vi "data_analysis main.vi"() -> ()   [LabVIEW 2017]
uses:
  <vilib>/Analysis/baseanly.llb/Mean (DBL).vi
  <vilib>/Waveform/WDTFileIO.llb/Export Waveforms To Spreadsheet File (1D).vi
  <vilib>/Utility/file.llb/Read Delimited Spreadsheet (DBL).vi
  <vilib>/Analysis/NI_AALBase.lvlib
panel:
  out "size(Zmag)":i32
  out "size(Z)":i32
  in  "停止":bool
  out "Zmag trajectory":waveform(dbl) caption="元素"
  out "Ext.":dbl
  out "Z pos":waveform(dbl)[](graph)
  out "Zmag pos":waveform(dbl)(graph)
  out "data name":string
  out "cursor pos":dbl
  out "cursor length":dbl
  out "zmag cursor pos":dbl
  out "zmag cursor length":dbl
  out "current bead":string
  in  "graphs":enum32{"raw data", "force calculation"}(tab)
  in  "next":bool
  out "XY图":cluster{dbl[], dbl[]}(graph)
  in  "ref NO.":i32 min=0
  in  "remove drift":bool
  in  "sample rate":dbl=200.0
  in  "zero point offset":bool
  out "x_0":dbl caption="X0" format="%0.2f"
  out "y_0":dbl caption="Y0" format="%0.2f"
  out "z_0":dbl caption="Z0" format="%0.2f"
  in  "file save path":path
  in  "数据另存为":bool
  in  "data type":enum16{"tdms", "gr", "excel"}(ring)
  out "保存完成？":bool
  in  "file path":path
  in  "load data":bool
  in  "data info":i32(listbox)
  in  "bead NO.":i32 min=0
  in  "trajectory":i32 min=0
  out "Z mag":dbl
  in  "zmag or force":enum32{"zmag", "force"}(radio)
  in  "load txt":bool
  out "data num":i32
  in  "Last":bool
  out "size(align)":i32
  in  "left rank":i32=10
  in  "right rank":i32=8
  in  "doubleFace?":bool
  in  "B":dbl=-1.436
  in  "A":dbl=142.6
  in  "cali source":enum32{"X", "Y"}(radio)
  out "Power spectrum (um^2/Hz)":cluster{dbl[], "Spectrum out":dbl[]}[](graph)
  in  "Z_shift":dbl
  out "Force graph":cluster{dbl[], dbl[]}(graph)
  in  "accept":bool
  in  "force estimate":bool
  in  "Fit settings":T1={"#PSD Averages"=40, "Correct camera acquisition artifacts"=TRUE, "Autorange"=TRUE, "fstart (Hz)"=0.0, "Pendulum geometry"=FALSE, "Fit model"=FALSE} {"#PSD Averages" min=1}
  in  "fsampling (Hz)":dbl=2800.0
  in  "DNA length (um)":dbl=0.658
  out "Fit Results":T2
  out "fit data":dbl[][](array[numeric])
  # "load force-zmag"
  # "F="
  # "exp(                *Zmag)"
  # "*"
  # "exp(                *Zmag)"
  # "+"
  # "*"
  # "Fit parameters"
  # "Calculated quantities"
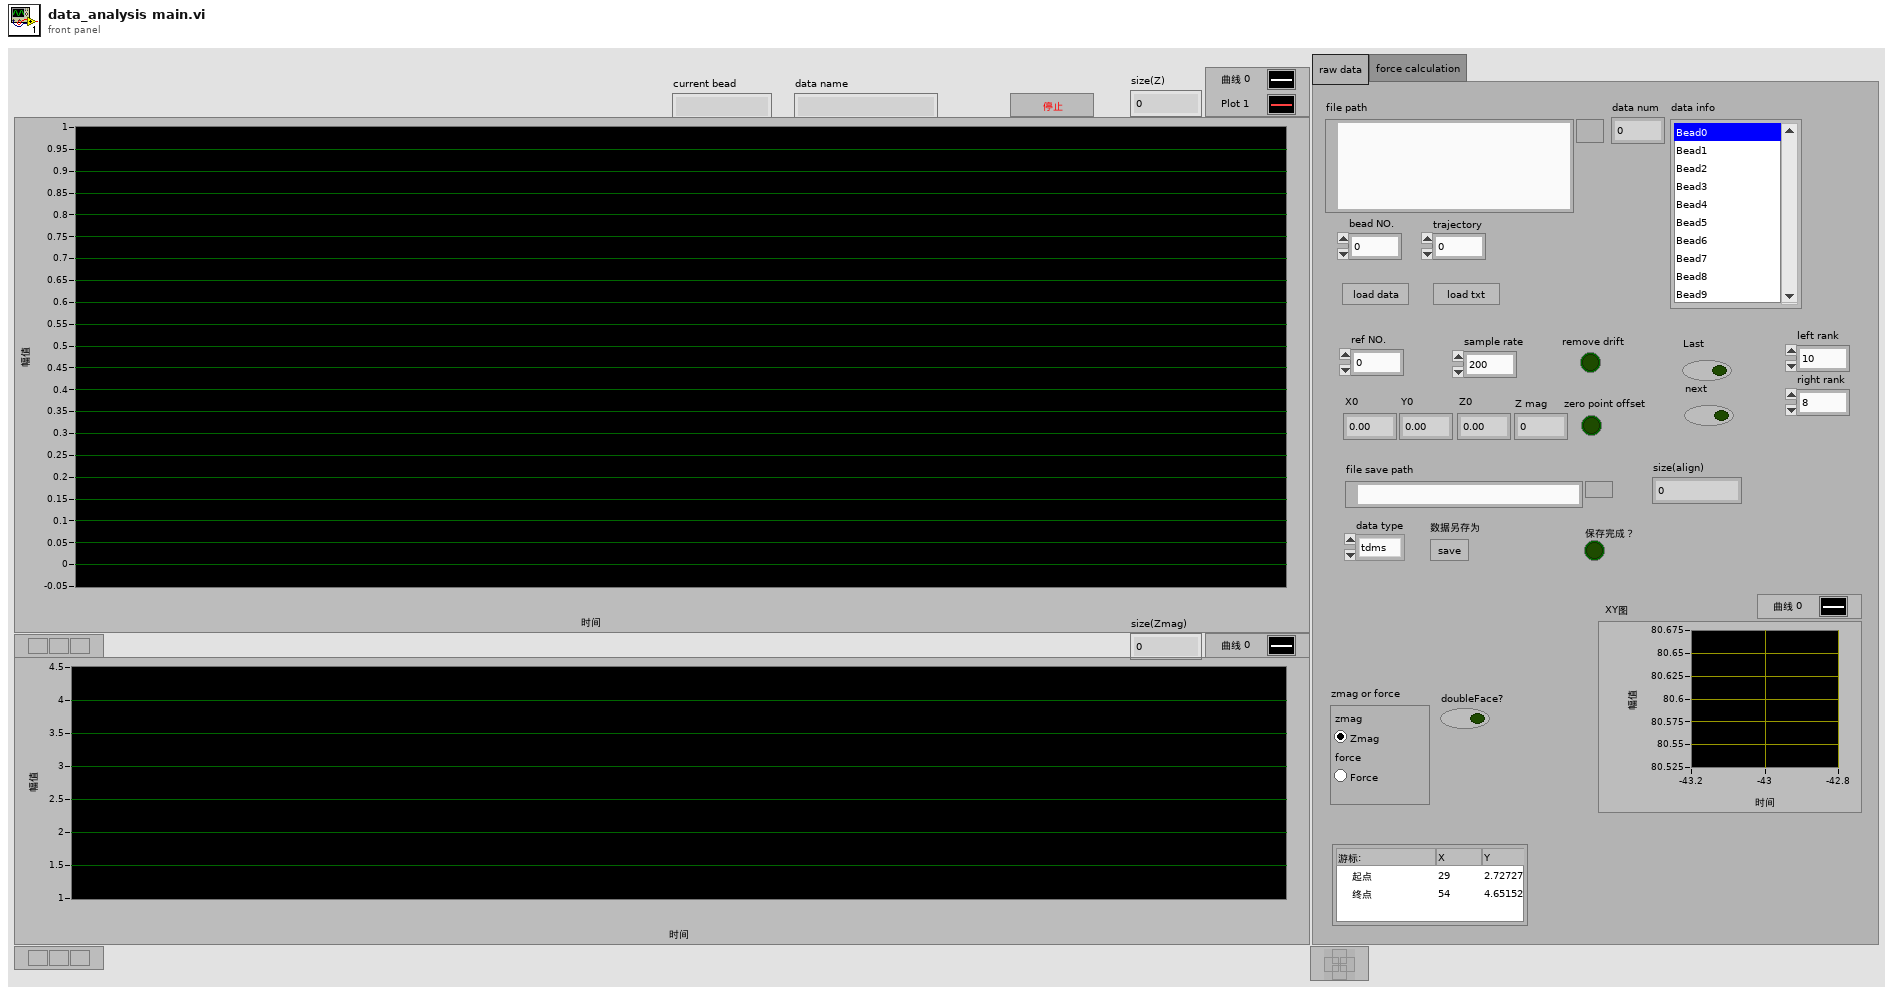
[diagram p1: front panel]
types:
  T1 = cluster{"#PSD Averages":u8, "Correct camera acquisition artifacts":bool, "Autorange":bool, "fstart (Hz)":dbl, "Pendulum geometry":bool, "Fit model":bool}
  T2 = cluster{"fcut (Hz)":dbl, "x2 (µm^2)":dbl, "Force (pN)":dbl, "Radius (µm)":dbl, "Apparent hydrodyn. radius (µm)":dbl, "fcut Error (Hz)":dbl, "x2 Error (µm^2)":dbl, "Force Error (pN)":dbl, "Radius Error (µm)":dbl, "Residue (unbiased)":dbl, "In range?":bool}
  T3 = enum16{"open", "open or create", "create or replace", "create", "open (read-only)"}
  T4 = enum16{"big-endian, network order", "native, host order", "little-endian"}
  T5 = enum16{"open", "replace", "create", "open or create", "replace or create", "replace or create with confirmation"}
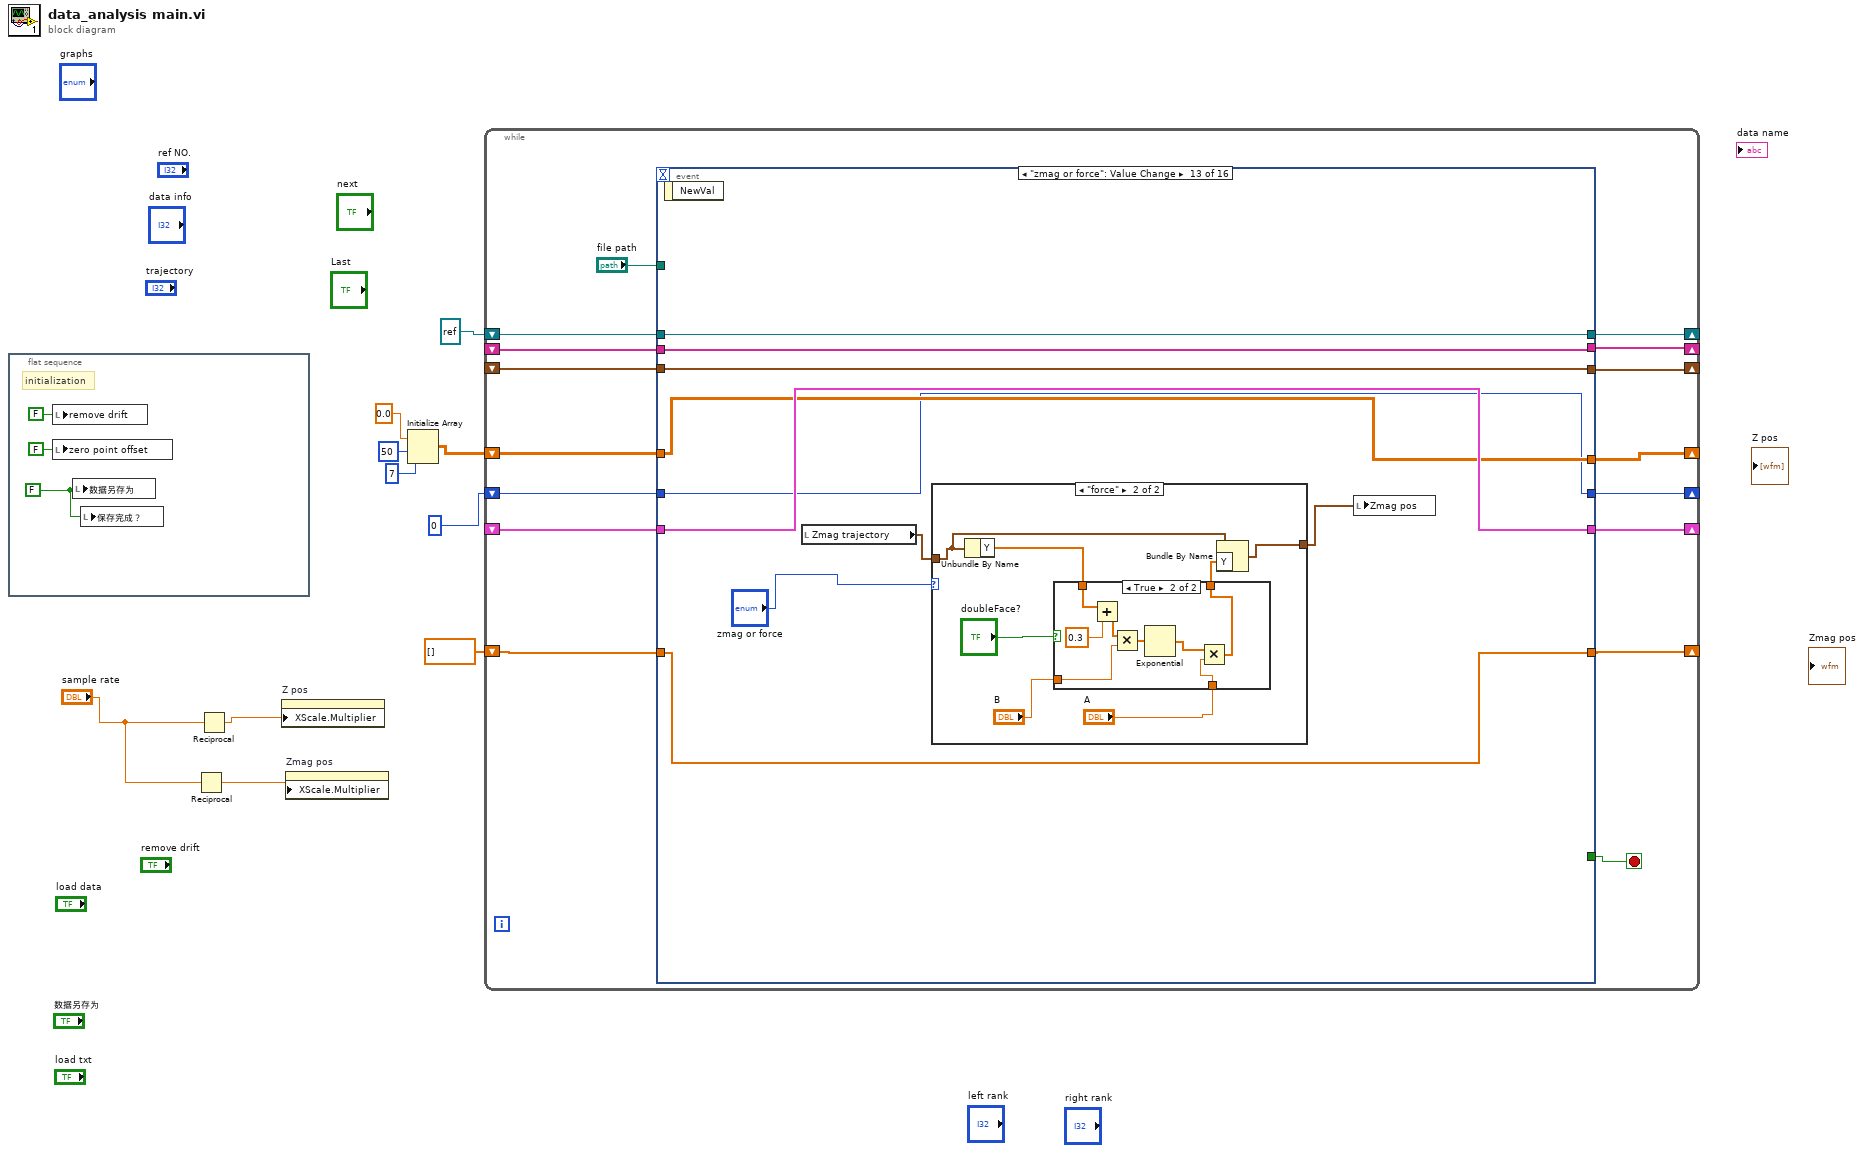
[diagram p0: block diagram]
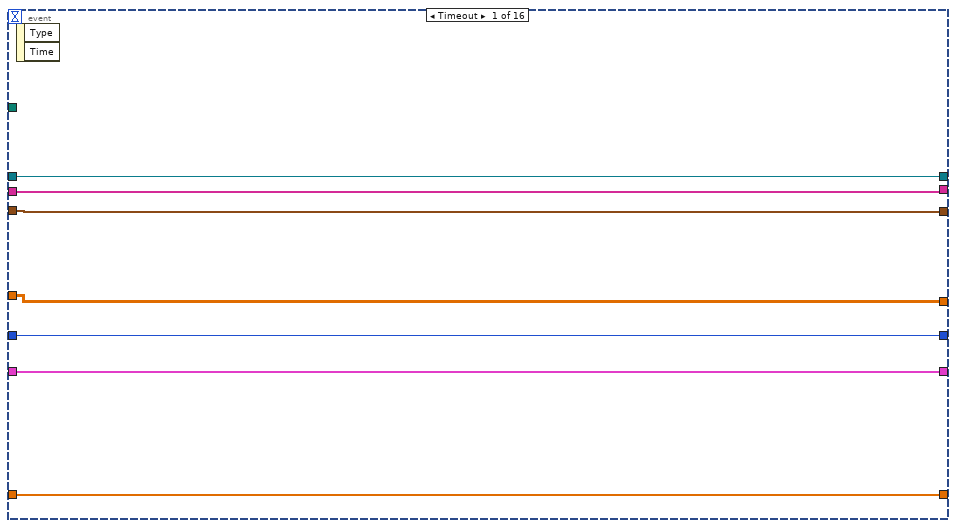
[diagram p2: hidden frame]
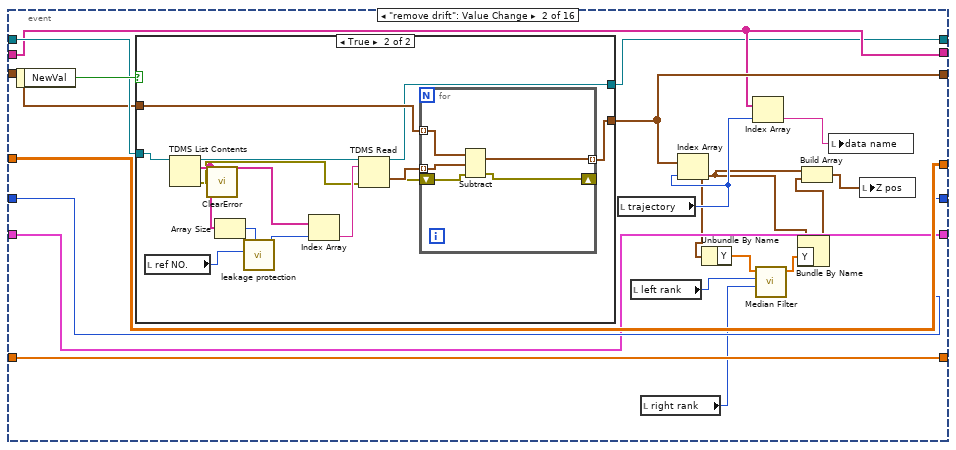
[diagram p3: hidden frame]
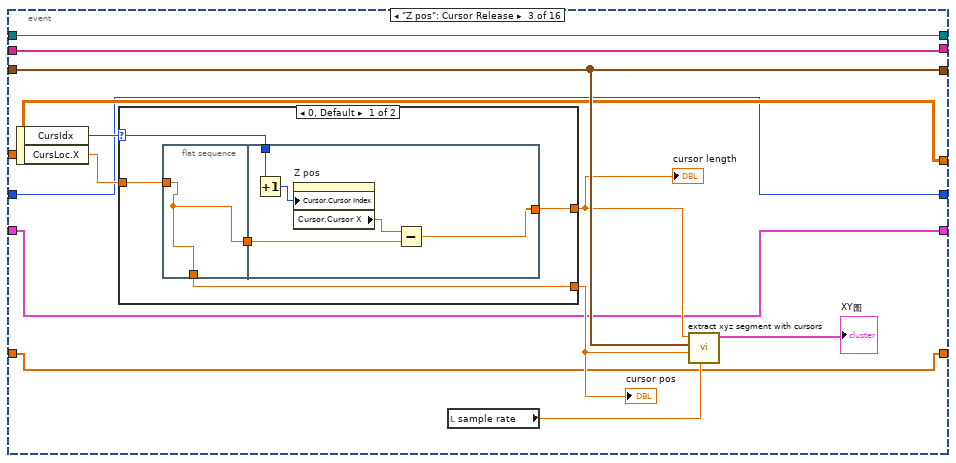
[diagram p5: hidden frame]
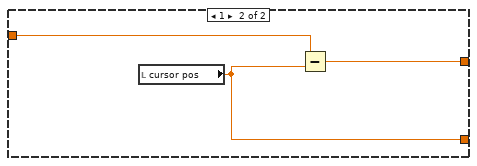
[diagram p6: hidden frame]
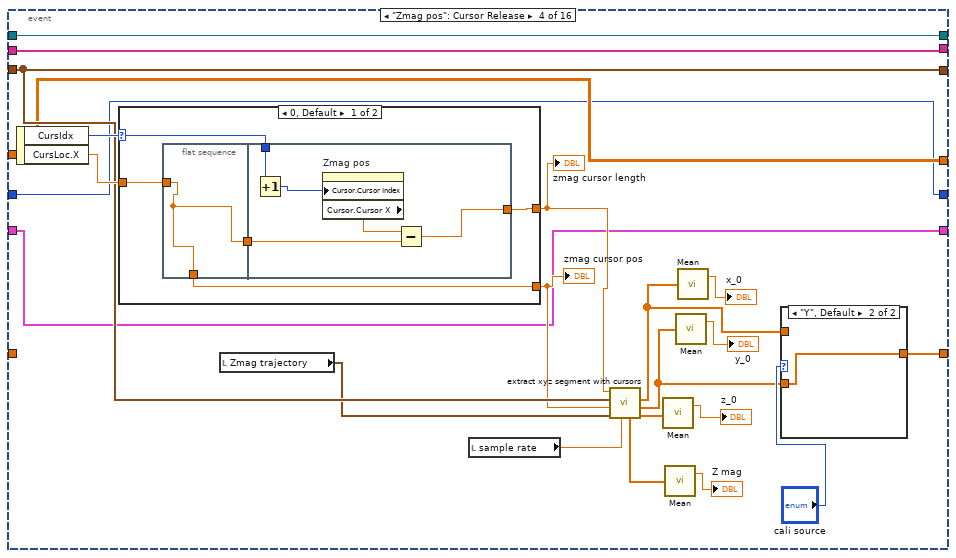
[diagram p7: hidden frame]
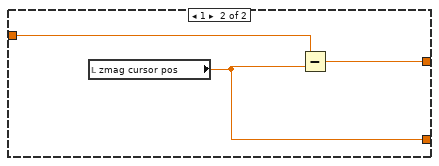
[diagram p9: hidden frame]
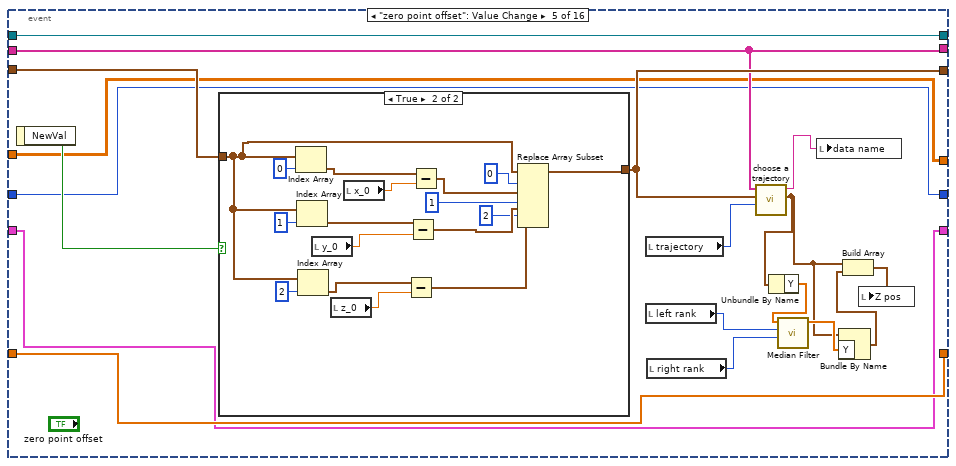
[diagram p10: hidden frame]
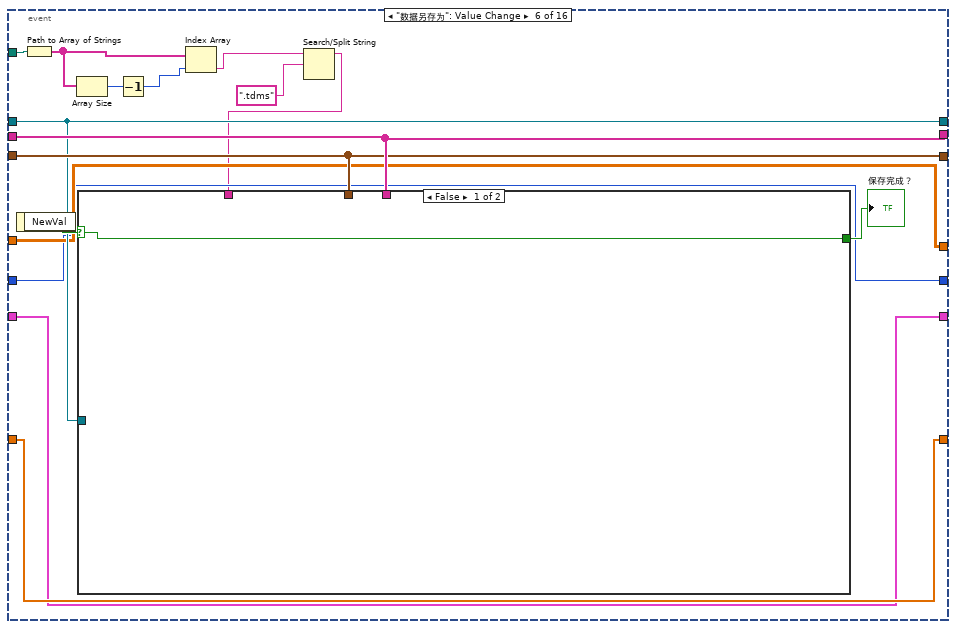
[diagram p12: hidden frame]
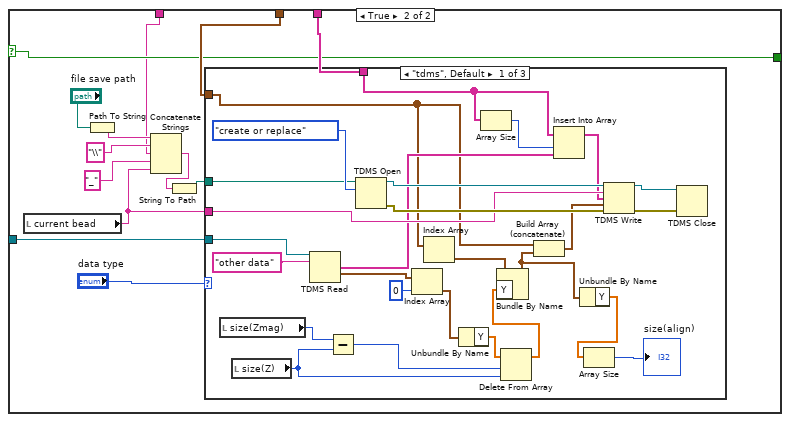
[diagram p13: hidden frame]
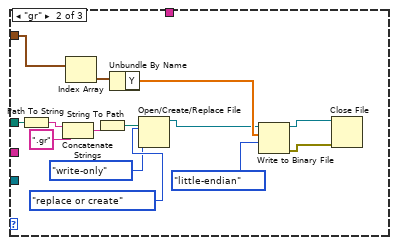
[diagram p14: hidden frame]
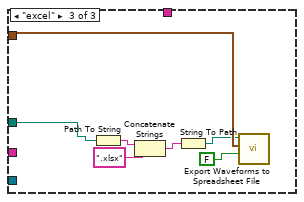
[diagram p15: hidden frame]
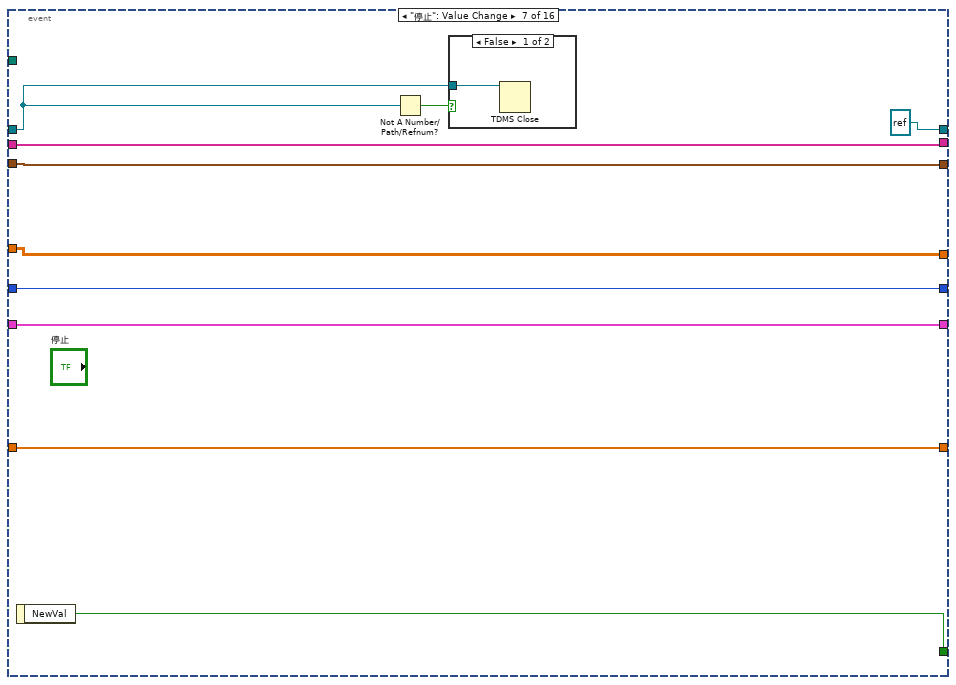
[diagram p16: hidden frame]
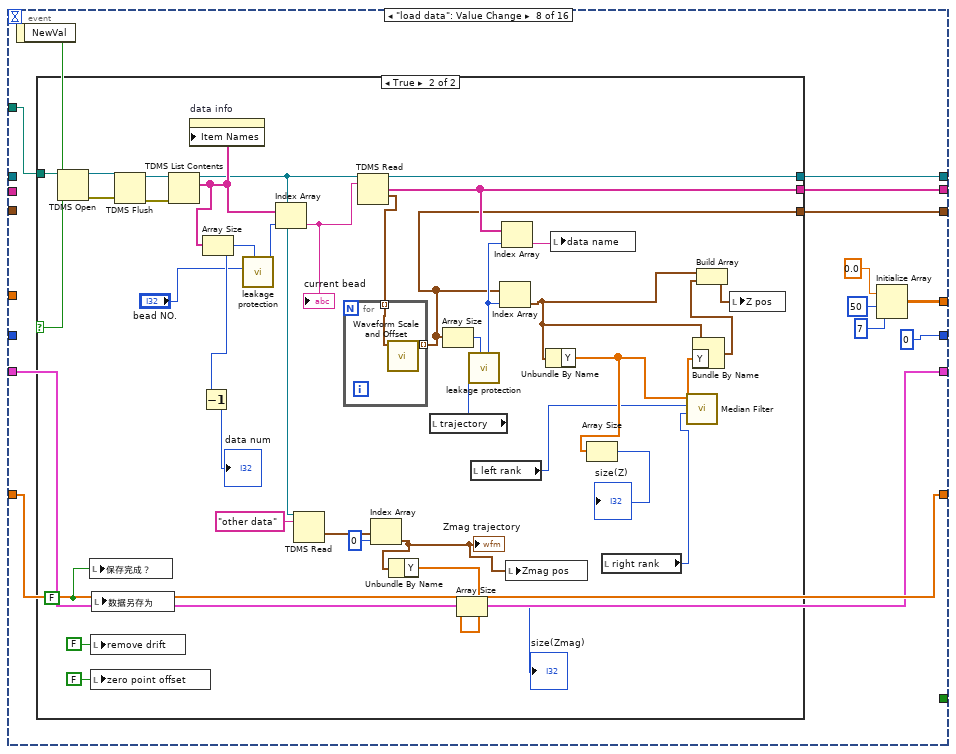
[diagram p18: hidden frame]
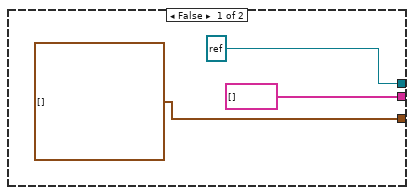
[diagram p19: hidden frame]
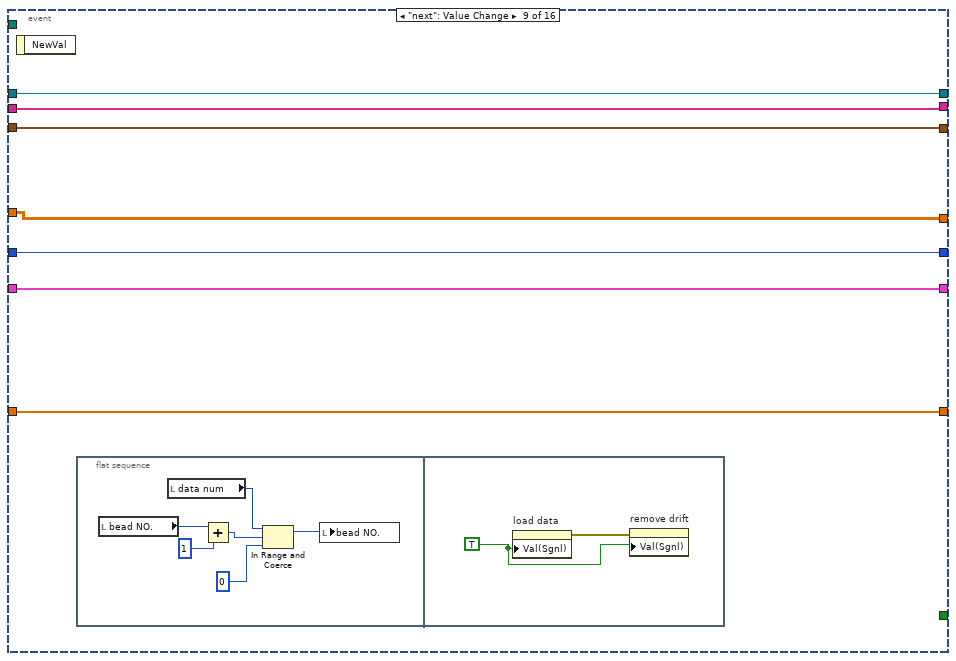
[diagram p20: hidden frame]
diagram:
  n1 = flat-sequence {
    frame #0 {
      w11 = FALSE ("数据另存为")
      # "initialization"
      n2 = local write "remove drift"(FALSE ("remove drift")) -> ()
      n3 = local write "zero point offset"(FALSE ("zero point offset")) -> ()
      n4 = local write "数据另存为"(w11) -> ()
      n5 = local write "保存完成？"(w11) -> ()
    }
  }
  n6 = Reciprocal(x="sample rate") -> (1/x=w1:dbl)
  n7 = Reciprocal(x="sample rate") -> (1/x=w3:dbl)
  n8 = property on="Z pos" class="WFGraph (strict)"("XScale.Multiplier"=w3) -> ()  [unwired: 2 in, 2 out]
  n9 = property on="Zmag pos" class="WFGraph (strict)"("XScale.Multiplier"=w1) -> ()  [unwired: 2 in, 2 out]
  n10 = Initialize Array(0.0 ("元素"), 50 ("维数大小"), 7 ("维数大小")) -> (w7:dbl[][])
  n11 = while {
    shift-right: [w27] -> _
    shift-left: refnum<k34> refnum ("tdms file out") -> [w22]
    shift-right: [w26] -> _
    shift-left: _ -> [w24]
    shift-right: [w25] -> _
    shift-left: _ -> [w23]
    shift-right: [w21] -> _
    shift-left: dbl[] [] ("Y") -> [w20]
    shift-right: [w19] -> _
    shift-left: _ -> [w18]
    shift-right: [w15] -> _
    shift-left: w7 -> [w17]
    shift-right: [w14] -> _
    shift-left: 0 -> [w16]
    stop <- w29 stop-if-true
    n12 = event "事件结构" shown="[12] \"zmag or force\": Value Change" {
      selector: _ -> [_ _ _ _ _ _ _ _ _ _ _ _ _ _ _ _]
      dyn-events: _ -> [_ _ _ _ _ _ _ _ _ _ _ _ _ _ _ _]
      timeout: _ -> [_ _ _ _ _ _ _ _ _ _ _ _ _ _ _ _]
      tunnel: [_ _ _ _ _ _ w265 _ _ _ _ _ _ _ _ _] -> w29
      tunnel: "file path" -> [_ _ _ _ _ w184 _ w278 _ _ w364 _ _ _ _ _]
      tunnel: [w34 w49 w81 w114 w153 w189 refnum<k34> refnum ("tdms file out") w277 w327 w342 w355 w406 w416 w457 refnum<k34> refnum ("tdms file out") w509] -> w27
      tunnel: [w36 w51 w89 w125 w155 w192 w264 w276 w326 w341 w352 w405 w415 w456 w495 w510] -> w26
      tunnel: [w35 w52 w86 w122 w156 w191 w263 w275 w325 w340 w354 w404 w414 w455 w494 w512] -> w25
      tunnel: w24 -> [w36 w51 w89 w125 w155 w192 w264 _ w326 w341 w351 w405 w415 w456 w495 w510]
      tunnel: w23 -> [w35 w53 w86 w122 w158 w191 w263 _ w325 w340 w353 w404 w414 w455 w494 w512]
      tunnel: w22 -> [w34 w54 w81 w114 w153 w189 w257 _ w327 w342 w355 w406 w416 w457 w487 w509]
      tunnel: [w32 w46 w79 w105 w151 w187 w261 w273 w324 w339 w362 w403 w413 w439 w491 w506] -> w21
      tunnel: w20 -> [w32 w46 w79 _ w151 w187 w261 w273 w324 w339 w362 w403 w413 w439 w491 w506]
      tunnel: [w30 w44 w77 w111 w149 w185 w259 w272 w323 w338 w361 w400 w412 w453 w489 w504] -> w19
      tunnel: w18 -> [w30 w44 w77 w111 w149 w185 w259 w272 w323 w338 w361 _ w412 w453 w489 w504]
      tunnel: w17 -> [w33 w47 w80 w113 w152 w188 w262 _ w322 w337 _ w392 w411 w452 w492 w507]
      tunnel: w16 -> [w31 w45 w78 w112 w150 w186 w260 _ w321 w336 _ w391 w410 w451 w490 w505]
      tunnel: [w33 w47 w80 w113 w152 w188 w262 w268 w322 w337 w357 w392 w411 w445 w492 w507] -> w15
      tunnel: [w31 w45 w78 w112 w150 w186 w260 0 w321 w336 0 w391 w410 w442 w490 w505] -> w14
      event Timeout {
        n13 = event-data() -> ()  [unwired: 1 in, 2 out]
      }
      event "remove drift": Value Change {
        n14 = event-data() -> ("NewVal"=w55:bool)  [unwired: 1 in]
        n15 = case shown="True" w55 {
          tunnel: w54 -> [w56 w66]
          tunnel: w53 -> [w57 w63]
          tunnel: [w57 w60] -> w52
          tunnel: [w56 w59] -> w49
          frame False {
          }
          frame True {
            n16 = local read "ref NO."() -> (w65:i32)
            n17 = TDMS List Contents(7:w66) -> (0:w58:errorcluster, 2:w69:string[], 3:w71:refnum<k34>)  [unwired: 2 in, 1 out]
            n18 = call <vilib>:"ClearError.vi"("error in (no error)"=w58) -> ("error out"=w64:errorcluster)
            n19 = Array Size(array=w69) -> (size(s)=w68:i32)
            n20 = call "leakage protection.vi"("matrix size"=w68, "index in"=w65) -> ("index out"=w67:i32)  [unwired: 9 in]
            n21 = Index Array(array=w69, index=w67) -> (element=w70:string)
            n22 = TDMS Read(0:w71, 5:w70, 11:w64) -> (4:w59:refnum<k34>, 10:w62:waveform(dbl)[], 15:w61:errorcluster)  [unwired: 5 in, 3 out]
            n23 = for {
              tunnel: w63 -> [w76] mode=indexing
              tunnel: w62 -> [w75] mode=indexing
              shift-right: [w73] -> _
              shift-left: w61 -> [w74]
              tunnel: [w72] -> w60 mode=indexing
              n24 = Subtract(1:w75, 2:w76, 4:w74) -> (0:w72:waveform(dbl), 3:w73:errorcluster)
            }
          }
        }
        n25 = local read "trajectory"() -> (w50:i32)
        n26 = local read "left rank"() -> (w38:i32)
        n27 = local read "right rank"() -> (w37:i32)
        n28 = Index Array(array=w52, index=w50) -> (element=w41:waveform(dbl))
        n29 = Unbundle By Name(w41) -> ("Y"=w42:dbl[])
        n30 = Index Array(array=w51, index=w50) -> (element=w48:string)
        n31 = call <vilib>:"Median Filter.vi"("right rank"=w37, "left rank"=w38, "X"=w42) -> ("Filtered X"=w43:dbl[])  [unwired: 7 in, 1 out]
        n32 = Bundle By Name(cluster=w41, "Y"=w43) -> (w40:waveform(dbl))
        n33 = Build Array(w41, w40) -> (w39:waveform(dbl)[])
        n34 = local write "data name"(w48) -> ()
        n35 = local write "Z pos"(w39) -> ()
      }
      event "Z pos": Cursor Release {
        n36 = event-data() -> ("CursIdx"=w88:i32, "CursLoc.X"=w87:dbl)  [unwired: 1 in]
        n37 = case shown="0, Default" w88 {
          selector: w88 -> [w93 _]
          tunnel: w87 -> [w94 w103]
          tunnel: [w91 w102] -> w84
          tunnel: [w90 w101] -> w85
          frame 0, Default {
            n38 = flat-sequence {
              tunnel: w94 -> [w95]
              tunnel: [w95] -> w92
              tunnel: [w95] -> w90
              tunnel: w93 -> [w99]
              tunnel: w92 -> [w97]
              tunnel: [w96] -> w91
              frame #0 {
              }
              frame #1 {
                n39 = Increment(x=w99) -> (x+1=w100:i32)
                n40 = property on="Z pos" class="WFGraph (strict)"("Cursor.Cursor Index"=w100) -> ("Cursor.Cursor X"=w98:dbl)  [unwired: 2 in, 2 out]
                n41 = Subtract(x=w98, y=w97) -> (x-y=w96:dbl)
              }
            }
          }
          frame 1 {
            n42 = local read "cursor pos"() -> (w101:dbl)
            n43 = Subtract(x=w103, y=w101) -> (x-y=w102:dbl)
          }
        }
        "cursor length" <- w84
        "cursor pos" <- w85
        n44 = local read "sample rate"() -> (w83:dbl)
        n45 = call "extract xyz segment with cursors.vi"("sample rate"=w83, "cursor pos"=w85, "data"=w86, "cursor length"=w84) -> ("xy cluster"=→"XY图":cluster{dbl[], dbl[]})  [unwired: 3 in, 4 out]
      }
      event "Zmag pos": Cursor Release {
        n46 = event-data() -> ("CursIdx"=w124:i32, "CursLoc.X"=w123:dbl)  [unwired: 1 in]
        n47 = case shown="0, Default" w124 {
          selector: w124 -> [w131 _]
          tunnel: w123 -> [w132 w141]
          tunnel: [w129 w140] -> w120
          tunnel: [w128 w139] -> w121
          frame 0, Default {
            n48 = flat-sequence {
              tunnel: w132 -> [w133]
              tunnel: [w133] -> w130
              tunnel: [w133] -> w128
              tunnel: w131 -> [w138]
              tunnel: w130 -> [w137]
              tunnel: [w136] -> w129
              frame #0 {
              }
              frame #1 {
                n49 = Increment(x=w138) -> (x+1=w134:i32)
                n50 = property on="Zmag pos" class="WFGraph (strict)"("Cursor.Cursor Index"=w134) -> ("Cursor.Cursor X"=w135:dbl)  [unwired: 2 in, 2 out]
                n51 = Subtract(x=w135, y=w137) -> (x-y=w136:dbl)
              }
            }
          }
          frame 1 {
            n52 = local read "zmag cursor pos"() -> (w139:dbl)
            n53 = Subtract(x=w141, y=w139) -> (x-y=w140:dbl)
          }
        }
        "zmag cursor length" <- w120
        "zmag cursor pos" <- w121
        n54 = local read "Zmag trajectory"() -> (w110:waveform(dbl))
        n55 = local read "sample rate"() -> (w119:dbl)
        n56 = call "extract xyz segment with cursors.vi"("sample rate"=w119, "Zmag trajectory"=w110, "cursor pos"=w121, "data"=w122, "cursor length"=w120) -> ("Z"=w118:dbl[], "Y"=w106:dbl[], "X"=w104:dbl[], "Z mag"=w109:dbl[])  [unwired: 2 in, 1 out]
        n57 = call-poly <vilib>:"Mean.vi"("X"=w118) -> ("mean"=→"z_0":dbl)  [unwired: 1 out]
        n58 = call-poly <vilib>:"Mean.vi"("X"=w109) -> ("mean"=→"Z mag":dbl)  [unwired: 1 out]
        n59 = call-poly <vilib>:"Mean.vi"("X"=w106) -> ("mean"=→"y_0":dbl)  [unwired: 1 out]
        n60 = call-poly <vilib>:"Mean.vi"("X"=w104) -> ("mean"=→"x_0":dbl)  [unwired: 1 out]
        n61 = case shown="\"Y\", Default" "cali source" {
          tunnel: w106 -> [_ w127]
          tunnel: [w126 w127] -> w105
          tunnel: w104 -> [w126 _]
          frame "X" {
          }
          frame "Y", Default {
          }
        }
      }
      event "zero point offset": Value Change {
        n62 = event-data() -> ("NewVal"=w159:bool)  [unwired: 1 in]
        n63 = case shown="True" w159 {
          tunnel: w158 -> [w160 w166]
          tunnel: [w160 w161] -> w156
          frame False {
          }
          frame True {
            n64 = Index Array(array=w166, index=0 ("索引")) -> (element=w174:waveform(dbl))
            n65 = Index Array(array=w166, index=1 ("索引")) -> (element=w172:waveform(dbl))
            n66 = Index Array(array=w166, index=2 ("索引")) -> (element=w170:waveform(dbl))
            n67 = local read "y_0"() -> (w171:dbl)
            n68 = local read "z_0"() -> (w169:dbl)
            n69 = local read "x_0"() -> (w173:dbl)
            n70 = Subtract(x=w170, y=w169) -> (x-y=w162:waveform(dbl))
            n71 = Subtract(x=w172, y=w171) -> (x-y=w164:waveform(dbl))
            n72 = Subtract(x=w174, y=w173) -> (x-y=w167:waveform(dbl))
            n73 = Replace Array Subset(array=w166, new element #1=w167, index #1=0 ("索引"), new element #2=w164, index #2=1 ("索引"), new element #3=w162, index #3=2 ("索引")) -> (w161:waveform(dbl)[])
          }
        }
        n74 = local read "trajectory"() -> (w157:i32)
        n75 = local read "left rank"() -> (w143:i32)
        n76 = local read "right rank"() -> (w142:i32)
        n77 = call "choose a trajectory.vi"("trajectory"=w157, "data"=w156, "bead info"=w155) -> ("trajectory"=w146:waveform(dbl), "data name"=w154:string)  [unwired: 7 in]
        n78 = Unbundle By Name(w146) -> ("Y"=w147:dbl[])
        n79 = call <vilib>:"Median Filter.vi"("right rank"=w142, "left rank"=w143, "X"=w147) -> ("Filtered X"=w148:dbl[])  [unwired: 7 in, 1 out]
        n80 = local write "data name"(w154) -> ()
        n81 = Bundle By Name(cluster=w146, "Y"=w148) -> (w145:waveform(dbl))
        n82 = Build Array(w146, w145) -> (w144:waveform(dbl)[])
        n83 = local write "Z pos"(w144) -> ()
      }
      event "数据另存为": Value Change {
        n84 = event-data() -> ("NewVal"=w193:bool)  [unwired: 1 in]
        n85 = Path to Array of Strings(0:w184) -> (2:w183:string[])  [unwired: 1 out]
        n86 = Array Size(array=w183) -> (size(s)=w182:i32)
        n87 = Decrement(x=w182) -> (x-1=w181:i32)
        n88 = Index Array(array=w183, index=w181) -> (element=w180:string)
        n89 = Search/Split String(string=w180, search string/char (-)=".tdms" ("搜索字符串/字符(-)")) -> (substring before match=w178:string)  [unwired: 1 in, 2 out]
        n90 = case shown="False" w193 {
          selector: w193 -> [w194 w199]
          tunnel: w192 -> [_ w207]
          tunnel: w191 -> [_ w206]
          tunnel: [w194 w199] -> w190
          tunnel: w189 -> [_ w198]
          tunnel: w178 -> [_ w197]
          frame False {
          }
          frame True {
            n91 = local read "current bead"() -> (w195:string)
            n92 = Path To String(path="file save path") -> (string=w204:string)
            n93 = Concatenate Strings(w204, "\\" ("字符串"), w197, "_" ("字符串"), w195) -> (w202:string)
            n94 = String To Path(string=w202) -> (path=w201:path)
            n95 = case shown="\"tdms\", Default" "data type" {
              tunnel: w207 -> [w222 _ _]
              tunnel: w206 -> [w209 w242 w255]
              tunnel: w201 -> [w231 w244 w253]
              tunnel: w195 -> [w228 _ _]
              tunnel: w198 -> [w224 _ _]
              frame "tdms", Default {
                n96 = local read "size(Zmag)"() -> (w217:i32)
                n97 = local read "size(Z)"() -> (w215:i32)
                n98 = TDMS Read(0:w224, 5:"other data" ("组名称输入")) -> (8:w221:string[], 10:w226:waveform(dbl)[])  [unwired: 6 in, 4 out]
                n99 = Subtract(x=w217, y=w215) -> (x-y=w216:i32)
                n100 = TDMS Open(10:T3."create or replace" ("操作(0:open)"), 11:w231) -> (0:w232:errorcluster, 3:w233:refnum<k34>)  [unwired: 5 in]
                n101 = Index Array(array=w226, index=0 ("索引")) -> (element=w212:waveform(dbl))
                n102 = Index Array(array=w209) -> (element=w208:waveform(dbl))  [unwired: 1 in]
                n103 = Unbundle By Name(w212) -> ("Y"=w218:dbl[])
                n104 = Array Size(array=w222) -> (size(s)=w219:i32)
                n105 = Delete From Array(array=w218, length=w216, index=w215) -> (array with subset deleted=w213:dbl[])  [unwired: 1 out]
                n106 = Bundle By Name(cluster=w208, "Y"=w213) -> (w211:waveform(dbl))
                n107 = Build Array (concatenate)(w209, w211) -> (w223:waveform(dbl)[])
                n108 = Insert Into Array(array=w222, index=w219, new element=w221) -> (w220:string[])
                n109 = Unbundle By Name(w211) -> ("Y"=w210:dbl[])
                n110 = Array Size(array=w210) -> (size(s)=→"size(align)":i32)
                n111 = TDMS Write(0:w233, 5:w228, 7:w220, 9:w223, 11:w232) -> (4:w230:refnum<k34>, 15:w229:errorcluster)  [unwired: 1 in, 2 out]
                n112 = TDMS Close(8:w229, 11:w230) -> ()  [unwired: 2 out]
              }
              frame "gr" {
                n113 = Path To String(path=w244) -> (string=w247:string)
                n114 = Concatenate Strings(w247, ".gr" ("字符串")) -> (w245:string)
                n115 = Index Array(array=w242) -> (element=w241:waveform(dbl))  [unwired: 1 in]
                n116 = String To Path(string=w245) -> (path=w243:path)
                n117 = Unbundle By Name(w241) -> ("Y"=w239:dbl[])
                n118 = Open/Create/Replace File(file path (use dialog)=w243, operation (0:open)=T5."replace or create" ("操作(0:open)"), access (0:read/write)=enum16{"read/write", "read-only", "write-only"}."write-only" ("权限(0:read/write)")) -> (refnum out=w238:refnum<file>)  [unwired: 3 in, 2 out]
                n119 = Write to Binary File(file (use dialog)=w238, data=w239, 9:T4."little-endian" ("字节顺序(0:big-endian, network order)")) -> (refnum out=w237:refnum<file>, error out=w236:errorcluster)  [unwired: 3 in, 1 out]
                n120 = Close File(refnum=w237, error in=w236) -> ()  [unwired: 2 out]
              }
              frame "excel" {
                n121 = Path To String(path=w253) -> (string=w252:string)
                n122 = Concatenate Strings(w252, ".xlsx" ("字符串")) -> (w250:string)
                n123 = String To Path(string=w250) -> (path=w249:path)
                n124 = call-poly <vilib>:"Export Waveforms to Spreadsheet File.vi"("multiple time columns? (single:F)"=FALSE ("append to file? (new file:F)"), "waveforms"=w255, "file path (dialog if empty)"=w249) -> ()  [unwired: 7 in, 2 out]
              }
            }
          }
        }
        "保存完成？" <- w190
      }
      event "停止": Value Change {
        n125 = event-data() -> ("NewVal"=w265:bool)  [unwired: 1 in]
        n126 = Not A Number/Path/Refnum?(number/path/refnum=w257) -> (NaN/Path/Refnum?=w258:bool)
        n127 = case shown="False" w258 {
          tunnel: w257 -> [w266 _]
          frame False {
            n128 = TDMS Close(11:w266) -> ()  [unwired: 1 in, 2 out]
          }
          frame True {
          }
        }
      }
      event "load data": Value Change {
        n129 = event-data() -> ("NewVal"=w274:bool)  [unwired: 1 in]
        n130 = case shown="True" w274 {
          tunnel: w278 -> [_ w318]
          tunnel: [refnum<k34> refnum ("tdms file out") w316] -> w277
          tunnel: [string[] [] ("channel name(s) out") w315] -> w276
          tunnel: [waveform(dbl)[] [] ("data") w293] -> w275
          frame False {
          }
          frame True {
            w296 = FALSE ("数据另存为")
            n131 = TDMS Open(11:w318) -> (0:w306:errorcluster, 3:w307:refnum<k34>)  [unwired: 6 in]
            n132 = local write "保存完成？"(w296) -> ()
            n133 = local write "remove drift"(FALSE ("remove drift")) -> ()
            n134 = local write "zero point offset"(FALSE ("zero point offset")) -> ()
            n135 = local write "数据另存为"(w296) -> ()
            n136 = TDMS Flush(4:w306, 7:w307) -> (0:w305:errorcluster, 3:w304:refnum<k34>)
            n137 = TDMS List Contents(4:w305, 7:w304) -> (2:w312:string[], 3:w303:refnum<k34>)  [unwired: 1 in, 2 out]
            n138 = property on="data info" class="LstBox (strict)"("Item Names"=w312) -> ()  [unwired: 2 in, 2 out]
            n139 = Array Size(array=w312) -> (size(s)=w311:i32)
            n140 = Decrement(x=w311) -> (x-1=→"data num":i32)
            n141 = call "leakage protection.vi"("matrix size"=w311, "index in"="bead NO.") -> ("index out"=w310:i32)  [unwired: 9 in]
            n142 = Index Array(array=w312, index=w310) -> (element=w317:string)
            "current bead" <- w317
            n143 = TDMS Read(0:w303, 5:"other data" ("组名称输入")) -> (10:w301:waveform(dbl)[])  [unwired: 6 in, 5 out]
            n144 = TDMS Read(0:w303, 5:w317) -> (4:w316:refnum<k34>, 8:w315:string[], 10:w294:waveform(dbl)[])  [unwired: 6 in, 3 out]
            n145 = for {
              tunnel: w294 -> [w320] mode=indexing
              tunnel: [w319] -> w293 mode=indexing
              n146 = call <vilib>:"Waveform Scale and Offset.vi"("waveform in"=w320) -> ("waveform out"=w319:waveform(dbl))  [unwired: 9 in, 1 out]
            }
            n147 = Index Array(array=w301, index=0 ("索引")) -> (element=w290:waveform(dbl))
            "Zmag trajectory" <- w290
            n148 = Unbundle By Name(w290) -> ("Y"=w289:dbl[])
            n149 = local read "trajectory"() -> (w309:i32)
            n150 = Array Size(array=w293) -> (size(s)=w313:i32)
            n151 = Array Size(array=w289) -> (size(s)=→"size(Zmag)":i32)
            n152 = call "leakage protection.vi"("matrix size"=w313, "index in"=w309) -> ("index out"=w314:i32)  [unwired: 9 in]
            n153 = local read "left rank"() -> (w283:i32)
            n154 = Index Array(array=w293, index=w314) -> (element=w286:waveform(dbl))
            n155 = Index Array(array=w315, index=w314) -> (element=w308:string)
            n156 = local write "Zmag pos"(w290) -> ()
            n157 = Unbundle By Name(w286) -> ("Y"=w288:dbl[])
            n158 = local write "data name"(w308) -> ()
            n159 = Array Size(array=w288) -> (size(s)=→"size(Z)":i32)
            n160 = local read "right rank"() -> (w282:i32)
            n161 = call <vilib>:"Median Filter.vi"("right rank"=w282, "left rank"=w283, "X"=w288) -> ("Filtered X"=w287:dbl[])  [unwired: 7 in, 1 out]
            n162 = Bundle By Name(cluster=w286, "Y"=w287) -> (w285:waveform(dbl))
            n163 = Build Array(w286, w285) -> (w284:waveform(dbl)[])
            n164 = local write "Z pos"(w284) -> ()
          }
        }
        n165 = Initialize Array(0.0 ("元素"), 50 ("维数大小"), 7 ("维数大小")) -> (w268:dbl[][])
      }
      event "next": Value Change {
        n166 = event-data() -> ()  [unwired: 1 in, 1 out]
        n167 = flat-sequence {
          frame #0 {
            n168 = local read "bead NO."() -> (w333:i32)
            n169 = local read "data num"() -> (w329:i32)
            n170 = Add(x=w333, y=1) -> (x+y=w331:i32)
            n171 = In Range and Coerce(upper limit=w329, x=w331, lower limit=0) -> (coerced(x)=w328:i32)  [unwired: 1 out]
            n172 = local write "bead NO."(w328) -> ()
          }
          frame #1 {
            w334 = TRUE
            n173 = property on="load data" class="Bool (strict)"("Val(Sgnl)"=w334) -> (error out=w335:errorcluster)  [unwired: 2 in, 1 out]
            n174 = property on="remove drift" class="Bool (strict)"(error in=w335, "Val(Sgnl)"=w334) -> ()  [unwired: 1 in, 2 out]
          }
        }
      }
      event "Last": Value Change {
        n175 = event-data() -> ()  [unwired: 1 in, 1 out]
        n176 = flat-sequence {
          frame #0 {
            n177 = local read "bead NO."() -> (w348:i32)
            n178 = local read "data num"() -> (w344:i32)
            n179 = Subtract(x=w348, y=1) -> (x-y=w346:i32)
            n180 = In Range and Coerce(upper limit=w344, x=w346, lower limit=0) -> (coerced(x)=w343:i32)  [unwired: 1 out]
            n181 = local write "bead NO."(w343) -> ()
          }
          frame #1 {
            w349 = TRUE
            n182 = property on="load data" class="Bool (strict)"("Val(Sgnl)"=w349) -> (error out=w350:errorcluster)  [unwired: 2 in, 1 out]
            n183 = property on="remove drift" class="Bool (strict)"(error in=w350, "Val(Sgnl)"=w349) -> ()  [unwired: 1 in, 2 out]
          }
        }
      }
      event "load txt": Value Change {
        n184 = event-data() -> ("NewVal"=w363:bool)  [unwired: 1 in]
        n185 = case shown="True" w363 {
          tunnel: w364 -> [_ w375]
          tunnel: [w366 w379] -> w354
          tunnel: w353 -> [w366 _]
          tunnel: [w365 string[] ["x", "y", "z", "zmag"] ("channel name(s) out")] -> w352
          tunnel: w351 -> [w365 _]
          frame False {
          }
          frame True {
            w380 = FALSE ("数据另存为")
            n186 = call-poly <vilib>:"Read Delimited Spreadsheet.vi"("file path (dialog if empty)"=w375) -> ("all rows"=w374:dbl[][])  [unwired: 9 in, 5 out]
            n187 = Transpose 2D Array(2D array=w374) -> (transposed array=w377:dbl[][])
            n188 = for {
              tunnel: w377 -> [w390] mode=indexing
              tunnel: [w388] -> w379 mode=indexing
              n189 = local read "sample rate"() -> (w387:dbl)
              n190 = Reciprocal(x=w387) -> (1/x=w389:dbl)
              n191 = Bundle By Name("Y"=w390) -> (w388:waveform(dbl))  [unwired: 1 in]
              n192 = call <vilib>:"Waveform Scale and Offset.vi"("scale"=w389, "waveform in"=w388) -> ()  [unwired: 8 in, 2 out]
            }
            n193 = local read "trajectory"() -> (w384:i32)
            n194 = local read "right rank"() -> (w367:i32)
            n195 = local read "left rank"() -> (w368:i32)
            n196 = local write "保存完成？"(w380) -> ()
            n197 = local write "remove drift"(FALSE ("remove drift")) -> ()
            n198 = local write "zero point offset"(FALSE ("zero point offset")) -> ()
            n199 = local write "数据另存为"(w380) -> ()
            n200 = Array Size(array=w379) -> (size(s)=w385:i32)
            n201 = call "leakage protection.vi"("matrix size"=w385, "index in"=w384) -> ("index out"=w386:i32)  [unwired: 9 in]
            n202 = Index Array(array=w379, index=w386) -> (element=w370:waveform(dbl))
            n203 = Unbundle By Name(w370) -> ("Y"=w373:dbl[])
            n204 = Index Array(array=w379, index=3 ("索引")) -> (element=w378:waveform(dbl))
            n205 = call <vilib>:"Median Filter.vi"("right rank"=w367, "left rank"=w368, "X"=w373) -> ("Filtered X"=w372:dbl[])  [unwired: 7 in, 1 out]
            n206 = local write "Zmag trajectory"(w378) -> ()
            n207 = Bundle By Name(cluster=w370, "Y"=w372) -> (w371:waveform(dbl))
            n208 = Build Array(w370, w371) -> (w369:waveform(dbl)[])
            n209 = local write "Zmag pos"(w378) -> ()
            n210 = local write "Z pos"(w369) -> ()
          }
        }
        n211 = Initialize Array(0.0 ("元素"), 50 ("维数大小"), 7 ("维数大小")) -> (w357:dbl[][])
      }
      event "force estimate": Value Change {
        n212 = event-data() -> ()  [unwired: 1 in, 1 out]
        n213 = local read "z_0"() -> (w395:dbl)
        n214 = Subtract(x="DNA length (um)", y="Z_shift") -> (x-y=w396:dbl)
        n215 = Add(x=w396, y=w395) -> (x+y=w394:dbl)
        "Ext." <- w394
        n216 = call "PSD fitting.vi"("DNA length (µm)"=w394, "fsampling (Hz)"="fsampling (Hz)", "Fit settings"="Fit settings", "X/Y data"=w403) -> ("Fit Results"=w400:T2, "Power spectrum (um^2/Hz)"=→"Power spectrum (um^2/Hz)":cluster{dbl[], "Spectrum out":dbl[]}[])  [unwired: 6 in]
        "Fit Results" <- w400
        n217 = local write "accept"(FALSE ("accept")) -> ()
      }
      event "zmag or force": Value Change {
        n218 = event-data() -> ()  [unwired: 1 in, 1 out]
        n219 = local read "Zmag trajectory"() -> (w408:waveform(dbl))
        n220 = case shown="\"force\"" "zmag or force" {
          tunnel: [w417 w423] -> w407
          tunnel: w408 -> [w417 w420]
          frame "zmag", Default {
          }
          frame "force" {
            n221 = Unbundle By Name(w420) -> ("Y"=w424:dbl[])
            n222 = case shown="True" "doubleFace?" {
              tunnel: w424 -> [w430 w433]
              tunnel: [w427 w431] -> w422
              tunnel: "B" -> [w426 w436]
              tunnel: "A" -> [w425 w435]
              frame False {
                n223 = Multiply(x=w430, y=w426) -> (x*y=w429:dbl[])
                n224 = Exponential(1:w429) -> (0:w428:dbl[])
                n225 = Multiply(x=w428, y=w425) -> (x*y=w427:dbl[])
              }
              frame True {
                n226 = Add(x=w433, y=0.3) -> (x+y=w434:dbl[])
                n227 = Multiply(x=w434, y=w436) -> (x*y=w438:dbl[])
                n228 = Exponential(1:w438) -> (0:w437:dbl[])
                n229 = Multiply(x=w437, y=w435) -> (x*y=w431:dbl[])
              }
            }
            n230 = Bundle By Name(cluster=w420, "Y"=w422) -> (w423:waveform(dbl))
          }
        }
        n231 = local write "Zmag pos"(w407) -> ()
      }
      event "accept": Value Change {
        n232 = event-data() -> ()  [unwired: 1 in, 1 out]
        n233 = case shown="True" "accept" {
          tunnel: w453 -> [_ w484]
          tunnel: w452 -> [w458 w470]
          tunnel: w451 -> [w459 w462]
          tunnel: [w458 w460] -> w445
          tunnel: [w459 w472] -> w442
          frame False {
          }
          frame True {
            n234 = Unbundle By Name(w484) -> ("Force (pN)"=w483:dbl, "Force Error (pN)"=w478:dbl, "Radius (µm)"=w477:dbl, "Radius Error (µm)"=w476:dbl, "fcut (Hz)"=w463:dbl)
            n235 = local read "Z mag"() -> (w466:dbl)
            n236 = local read "Ext."() -> (w468:dbl)
            n237 = Replace Array Subset(array=w470, new element=w468, index (row)=w462, index (col)=0 ("禁用的索引 (列)")) -> (w469:dbl[][])
            n238 = Replace Array Subset(array=w469, new element=w483, index (row)=w462, index (col)=1 ("禁用的索引 (列)")) -> (w475:dbl[][])
            n239 = Replace Array Subset(array=w475, new element=w478, index (row)=w462, index (col)=2 ("禁用的索引 (列)")) -> (w474:dbl[][])
            n240 = Replace Array Subset(array=w474, new element=w477, index (row)=w462, index (col)=3 ("禁用的索引 (列)")) -> (w473:dbl[][])
            n241 = Replace Array Subset(array=w473, new element=w476, index (row)=w462, index (col)=4 ("禁用的索引 (列)")) -> (w465:dbl[][])
            n242 = Replace Array Subset(array=w465, new element=w466, index (row)=w462, index (col)=5 ("禁用的索引 (列)")) -> (w461:dbl[][])
            n243 = Replace Array Subset(array=w461, new element=w463, index (row)=w462, index (col)=6 ("禁用的索引 (列)")) -> (w460:dbl[][])
            n244 = Increment(x=w462) -> (x+1=w472:i32)
          }
        }
        n245 = Array Subset(array=w445, index (row)=0 ("索引"), length (row)=w442, index (col)=0 ("索引"), length (col)=7 ("长度")) -> (w440:dbl[][])
        "fit data" <- w440
        n246 = Index Array(array=w440, index (col) #1=0 ("禁用的索引 (列)"), index (col) #2=1 ("索引 (列)")) -> (element #1=w449:dbl[], element #2=w447:dbl[])  [unwired: 2 in]
        n247 = Bundle(w449, w447) -> (→"Force graph":cluster{dbl[], dbl[]})  [unwired: 1 in]
      }
      event "file path": Value Change {
        n248 = event-data() -> ("NewVal"=w493:path)  [unwired: 1 in, 4 out]
        n249 = local write "file path"(w493) -> ()
        n250 = local write "bead NO."(0 ("bead NO.")) -> ()
        n251 = Not A Number/Path/Refnum?(number/path/refnum=w487) -> (NaN/Path/Refnum?=w486:bool)
        n252 = case shown="True" w486 {
          tunnel: w487 -> [w496 _]
          frame False {
            n253 = TDMS Close(11:w496) -> ()  [unwired: 1 in, 2 out]
          }
          frame True {
          }
        }
      }
      event "trajectory": Value Change {
        n254 = event-data() -> ("NewVal"=w511:i32)  [unwired: 1 in]
        n255 = call "choose a trajectory.vi"("trajectory"=w511, "data"=w512, "bead info"=w510) -> ("trajectory"=w501:waveform(dbl), "data name"=w508:string)  [unwired: 7 in]
        n256 = local read "left rank"() -> (w498:i32)
        n257 = Unbundle By Name(w501) -> ("Y"=w502:dbl[])
        n258 = local write "data name"(w508) -> ()
        n259 = local read "right rank"() -> (w497:i32)
        n260 = call <vilib>:"Median Filter.vi"("right rank"=w497, "left rank"=w498, "X"=w502) -> ("Filtered X"=w503:dbl[])  [unwired: 7 in, 1 out]
        n261 = Bundle By Name(cluster=w501, "Y"=w503) -> (w500:waveform(dbl))
        n262 = Build Array(w501, w500) -> (w499:waveform(dbl)[])
        n263 = local write "Z pos"(w499) -> ()
      }
    }
  }
